vi "Read Stop Bits.vi"(8 "error in (no error)":errorcluster, 11 "ElectrometerConfiguration in":refnum<class "ElectrometerConfiguration.lvclass">) -> (0 "error out":errorcluster, 2 "Stop Bits":u16(ring)=10 items=["1.0"=10, "1.5"=15, "2.0"=20], 3 "ElectrometerConfiguration out":refnum<class "ElectrometerConfiguration.lvclass">)   [LabVIEW 2016, in "ElectrometerConfiguration.lvclass"]
uses:
  ElectrometerConfiguration.lvclass
  ElectrometerConfiguration.lvclass/ElectrometerConfiguration.ctl
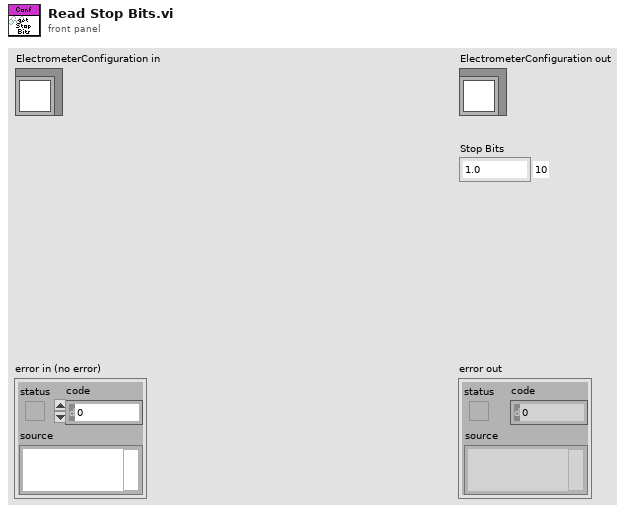
[diagram p1: front panel]
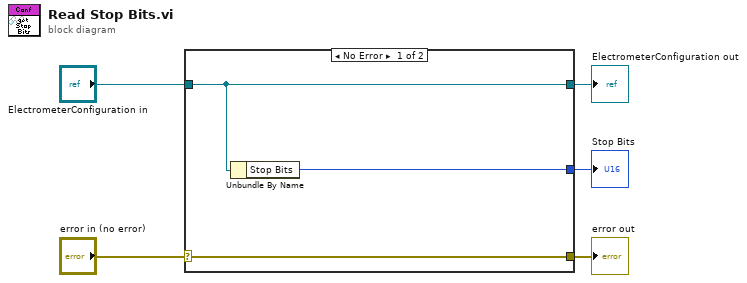
[diagram p0: block diagram]
diagram:
  n1 = case shown="No Error" "error in (no error)" {
    selector: "error in (no error)" -> [w8 w9]
    tunnel: [w8 w9] -> w4
    tunnel: [w7 w10] -> w2
    tunnel: "ElectrometerConfiguration in" -> [w7 w10]
    tunnel: [w6 _] -> w1
    frame No Error {
      n2 = Unbundle By Name(w7) -> ("Stop Bits"=w6:u16)
    }
    frame Error {
    }
  }
  "error out" <- w4
  "ElectrometerConfiguration out" <- w2
  "Stop Bits" <- w1
